vi "rdb_net_read_null.vi"(6 "timeout ms (10000)":i32=10000, 8 "error in (no error)":errorcluster, 11 "conn in":refnum<k5>) -> (0 "error out":errorcluster, 2 "data out":string, 3 "conn out":refnum<k5>)   [LabVIEW 2017]
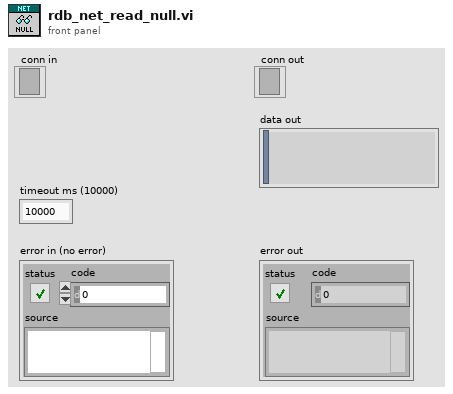
[diagram p1: front panel]
types:
  T1 = enum16{"Standard", "Buffered", "CRLF", "Immediate"}
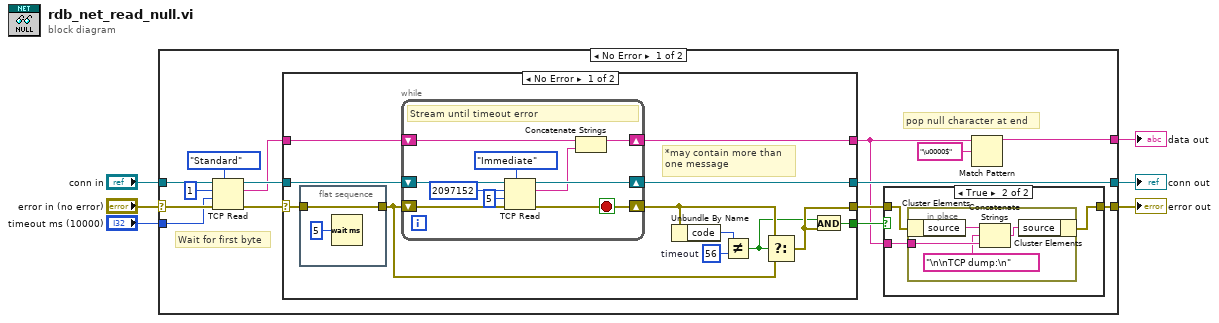
[diagram p0: block diagram]
diagram:
  n1 = case shown="No Error" "error in (no error)" {
    selector: "error in (no error)" -> [w20 w58]
    tunnel: "conn in" -> [w21 w57]
    tunnel: "timeout ms (10000)" -> [w19 _]
    tunnel: [w12 w58] -> w3
    tunnel: [w15 w57] -> w2
    tunnel: [w8 _] -> w1
    frame No Error {
      # "pop null character at end"
      # "Wait for first byte"
      n2 = TCP Read(connection ID=w21, bytes to read=1, error in (no error)=w20, 7:T1."Standard" ("mode (standard)"), 9:w19) -> (connection ID out=w14:refnum<k5>, data out=w13:string, error out=w16:errorcluster)
      n3 = case shown="No Error" w16 {
        selector: w16 -> [w33 w48]
        tunnel: [w24 w48] -> w11
        tunnel: [w31 w47] -> w15
        tunnel: w14 -> [w32 w47]
        tunnel: w13 -> [w30 w46]
        tunnel: [w29 w46] -> w7
        tunnel: [w22 _] -> w10
        frame No Error {
          w27 = 56  # timeout
          # "*may contain more than\none message"
          n4 = flat-sequence {
            tunnel: [w44] -> w25
            tunnel: w33 -> [w44]
            frame #0 {
              n5 = Wait (ms)(milliseconds to wait=u32 5) -> ()  [unwired: 1 out]
            }
          }
          n6 = while {
            shift-right: [w35] -> w26
            shift-left: w25 -> [w43]
            shift-right: [w41] -> w31
            shift-left: w32 -> [w42]
            shift-right: [w34] -> w29
            shift-left: w30 -> [w37]
            stop <- w35 stop-if-true
            # "Stream until timeout error"
            n7 = TCP Read(connection ID=w42, bytes to read=2097152, error in (no error)=w43, 7:T1."Immediate" ("mode (standard)"), 9:5 ("timeout ms (25000)")) -> (connection ID out=w41:refnum<k5>, data out=w36:string, error out=w35:errorcluster)
            n8 = Concatenate Strings(w37, w36) -> (w34:string)
          }
          n9 = Unbundle By Name(w26) -> ("code"=w28:i32)
          n10 = Not Equal?(x=w28, y=w27) -> (x != y?=w23:bool)
          n11 = Select(t=w26, s=w23, f=w25) -> (s? t:f=w24:errorcluster)
          n12 = And(x=w23, y=w24) -> (x .and. y?=w22:bool)
        }
        frame Error {
        }
      }
      n13 = case shown="True" w10 {
        tunnel: w7 -> [_ w52]
        tunnel: [w49 w51] -> w12
        tunnel: w11 -> [w49 w50]
        frame False {
        }
        frame True {
          n14 = in-place {
            in-place-border: w52 -> [w54]
            n15 = in-place-cluster #1(w50) -> ("source"=w56:string)
            n16 = Concatenate Strings(w56, "\n\nTCP dump:\n" ("format string"), w54) -> (w55:string)
            n17 = in-place-cluster #1("source"=w55) -> (w51:errorcluster)
          }
        }
      }
      n18 = Match Pattern(string=w7, regular expression="\u0000$") -> (before substring=w8:string)  [unwired: 1 in, 3 out]
    }
    frame Error {
    }
  }
  "error out" <- w3
  "conn out" <- w2
  "data out" <- w1
